vi "PQsendQueryPrepared.vi"(1 "paramLengths":i32, 2 "resultFormat":i32, 5 "stmtName":string, 7 "nParams":i32, 9 "paramValues":cluster{"const_char":string}, 11 "error in (no error)":errorcluster, 12 "paramFormats":i32) -> (6 "PQsendQueryPrepared":u32, 15 "error out":errorcluster)   [LabVIEW 2019, in "libpqlv.lvlib"]
uses:
  libpqlv.lvlib
  libpq.dll
panel:
  in  "conn":u32
  out "conn_out":u32
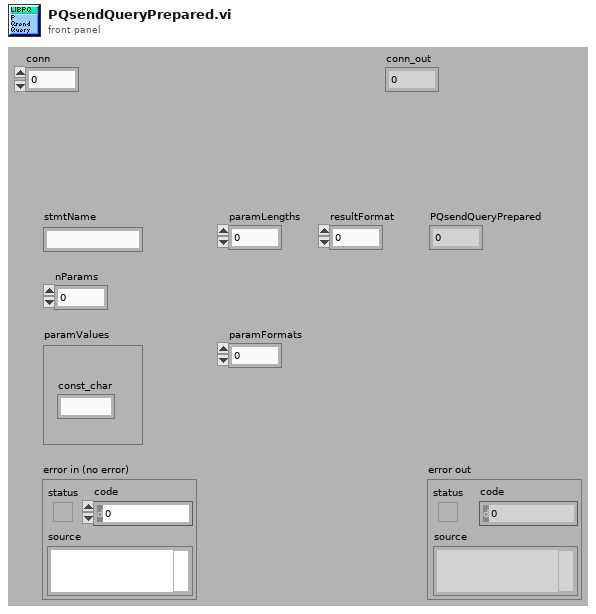
[diagram p1: front panel]
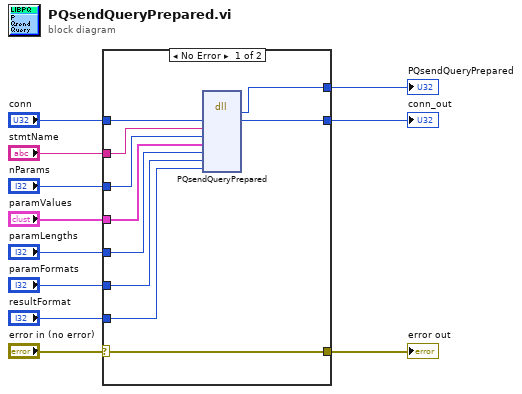
[diagram p0: block diagram]
diagram:
  n1 = case shown="No Error" "error in (no error)" {
    selector: "error in (no error)" -> [w21 w23]
    tunnel: [w21 w23] -> w10
    tunnel: [w20 _] -> w9
    tunnel: [w19 w22] -> w2
    tunnel: "stmtName" -> [w18 _]
    tunnel: "nParams" -> [w17 _]
    tunnel: "paramValues" -> [w12 _]
    tunnel: "paramLengths" -> [w16 _]
    tunnel: "paramFormats" -> [w15 _]
    tunnel: "resultFormat" -> [w14 _]
    tunnel: "conn" -> [w13 w22]
    frame No Error {
      n2 = dll-call lib="libpq.*" fn="PQsendQueryPrepared"("conn"=w13, "stmtName"=w18, "nParams"=w17, "paramValues"=w12, "paramLengths"=w16, "paramFormats"=w15, "resultFormat"=w14) -> ("PQsendQueryPrepared"=w20:u32, "conn"=w19:u32)  [unwired: 9 in, 2 out]
    }
    frame Error {
    }
  }
  "PQsendQueryPrepared" <- w9
  "error out" <- w10
  "conn_out" <- w2
